vi "Laser Rough Cutting.vi"(0 "configuration file path":path caption="production information", 1 "rough cutting msic":T1) -> ()   [LabVIEW 2018]
uses:
  Ctl.xio/rough cutting msic ctl.ctl
  SubVIS.xio/DataSocket/DataSocket_Tags.ctl
  Ctl.xio/part type.ctl
  SubVIS.xio/Creat Write List VI's/DefCtrl/Station.ctl
  <vilib>/Utility/file.llb/Read From Spreadsheet File (string).vi
  SubVIS.xio/DataSocket/Write PLC Vars/Write Bool Var in.vi
  SubVIS.xio/DataSocket/Read PLC Vars/Read String Var.vi
  SubVIS.xio/DataSocket/Write PLC Vars/Write String Var in.vi
  SubVIS.xio/DataSocket/Write PLC Vars/Write Dbl Var in.vi
  SubVIS.xio/DataSocket/Read PLC Vars/Read Bool Var.vi
panel:
  out "error out 2":errorcluster caption="error out"
  in  "SQL information":string
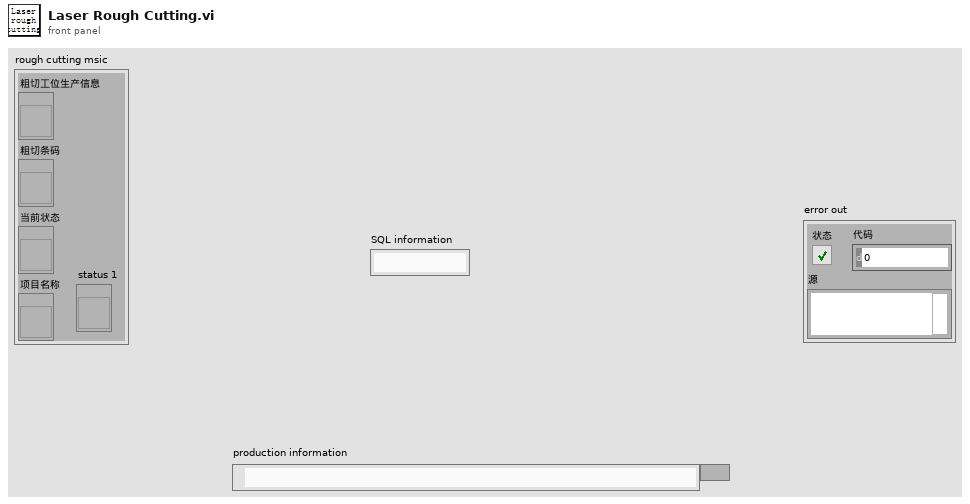
[diagram p1: front panel]
types:
  T1 = cluster{"粗切工位生产信息":refnum<vi>, "粗切条码":refnum<vi>, "当前状态":refnum<vi>, "项目名称":refnum<vi>, "status 1":refnum<vi>}
  T2 = typedef "Station.ctl" = enum16{"粗切工位", "热处理工位", "精切工位", "PDF焊接工位", "打凹点预载力工位", "收卷工位", "EOL工位"}
  T3 = typedef "rough cutting msic ctl.ctl" = cluster{"configuration file path":path, "DsOut":T4[], "scanner coms or ip":string, "BarCode":string, "scanner resource name out":refnum<visa-resource-name>, "Hopper car information":cluster{"Hopper car code":string, "Hopper car No":string, "plate No":string}, "pallet.produced number":i32, "SQL information":string, "Database":string[], "Serial number":i32, "database path":path, "rough cutting msic":cluster{"production info":refnum<vi>, "code":refnum<vi>, "status":refnum<vi>, "part type":refnum<vi>, "status":refnum<vi>}, "Part type":T5, "scanner ip ID":refnum<k5>, "Number of scans ":u8, "Incoming code":string, "Cut file":string, "Process code":string}
  T4 = typedef "DataSocket_Tags.ctl" = cluster{"Ds ID":refnum<k13>, "Tag":string}
  T5 = typedef "part type.ctl" = cluster{"Part type":string, "Material code":string, "Part number":string, "Supplier code":string, "Line code":string, "Customer code":string, "Color code":string, "Upper limit":i32, "Temperature":string, "Tot time":string, "EOL stations":string}
  T6 = cluster{"Hopper car code":string, "Hopper car No":string, "plate No":string}
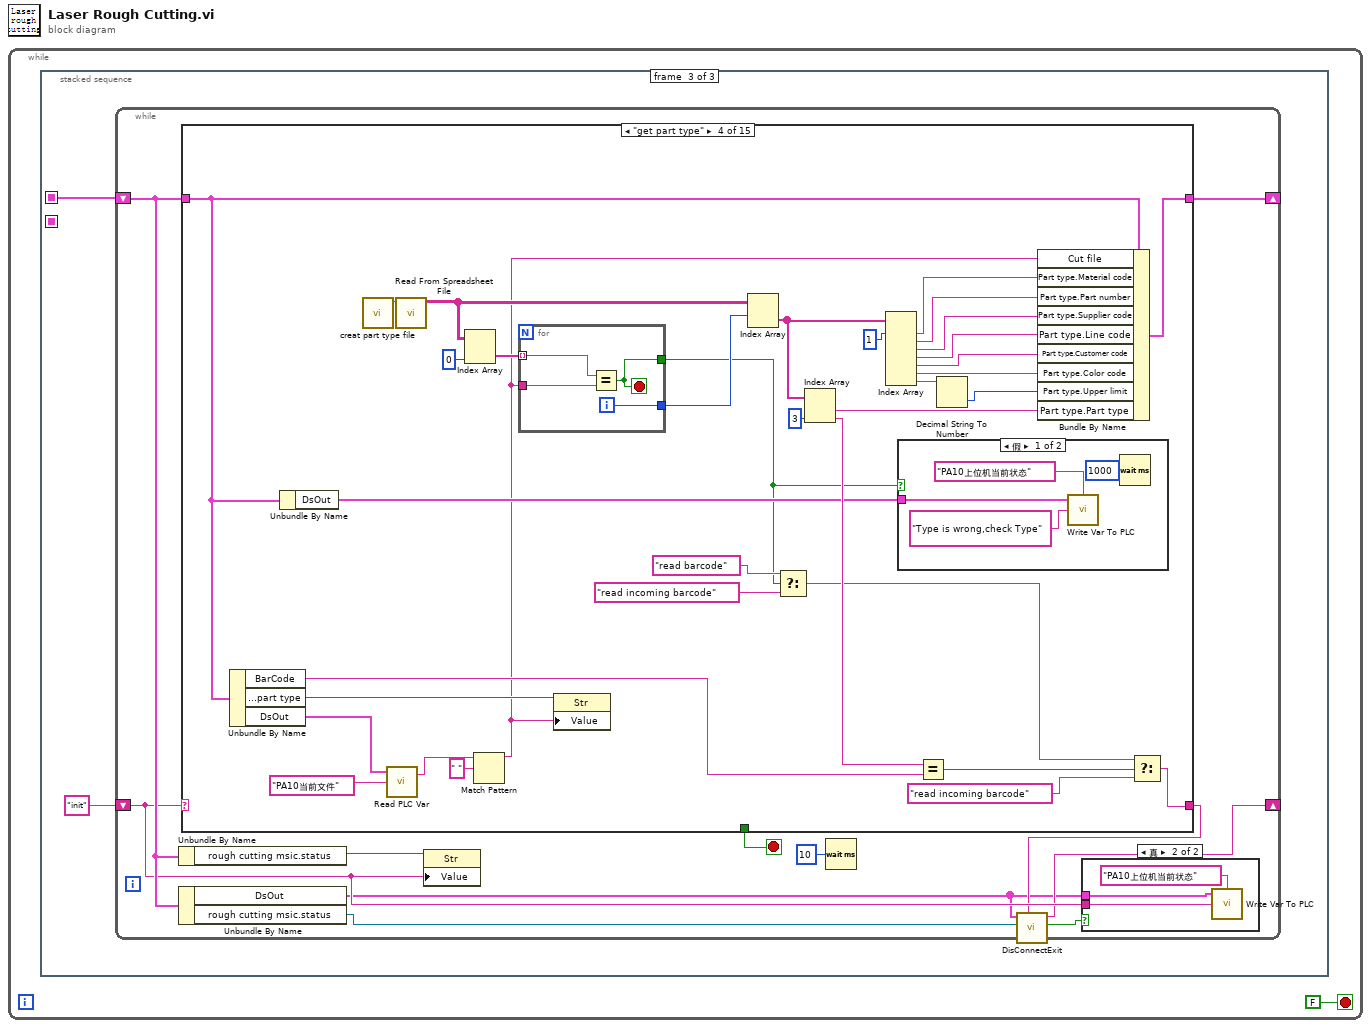
[diagram p0: block diagram]
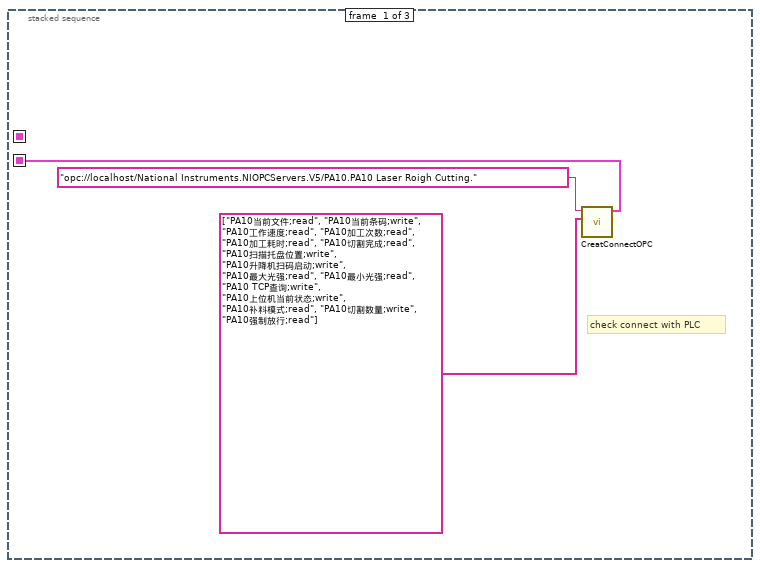
[diagram p2: hidden frame]
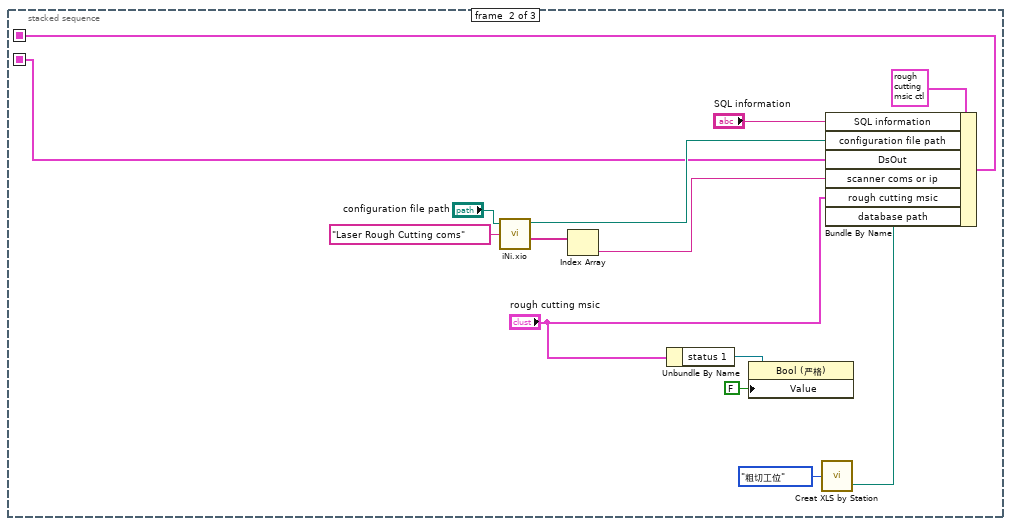
[diagram p3: hidden frame]
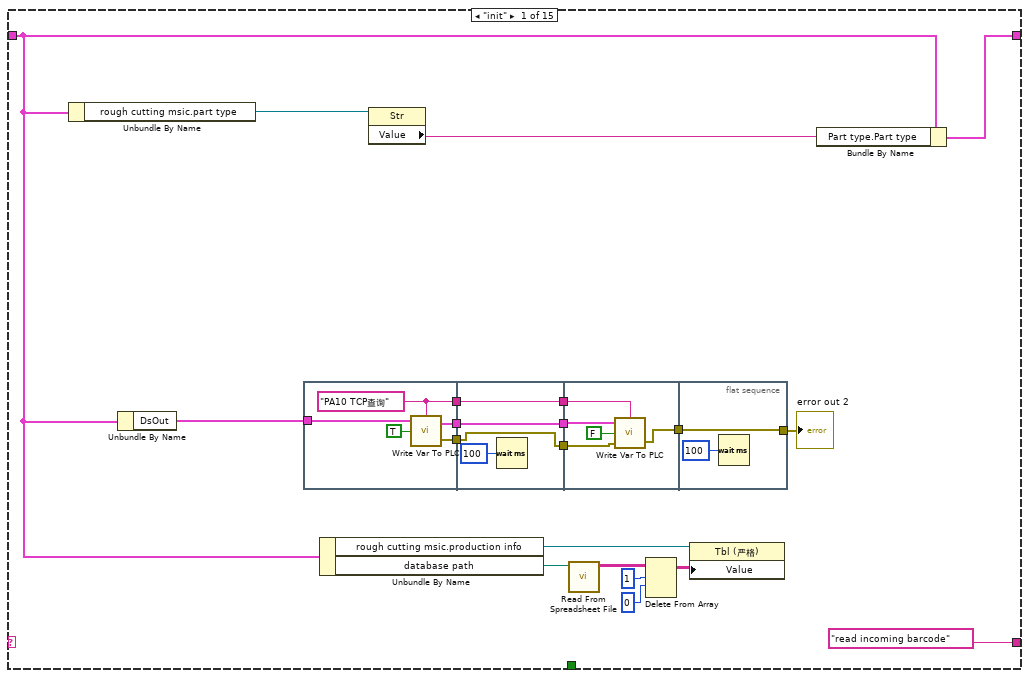
[diagram p5: hidden frame]
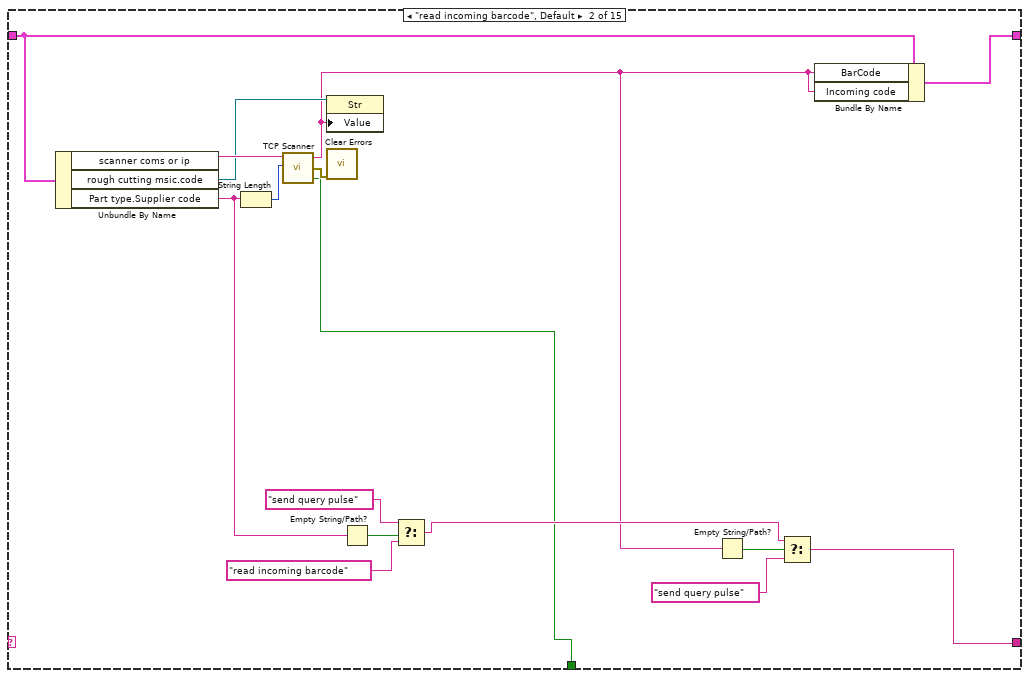
[diagram p6: hidden frame]
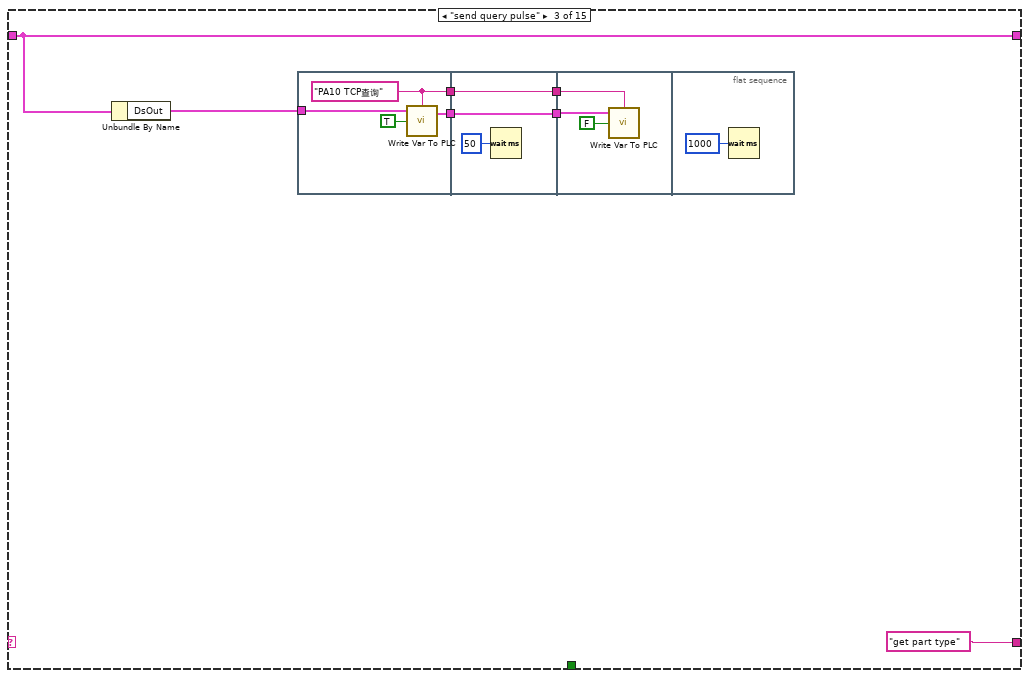
[diagram p7: hidden frame]
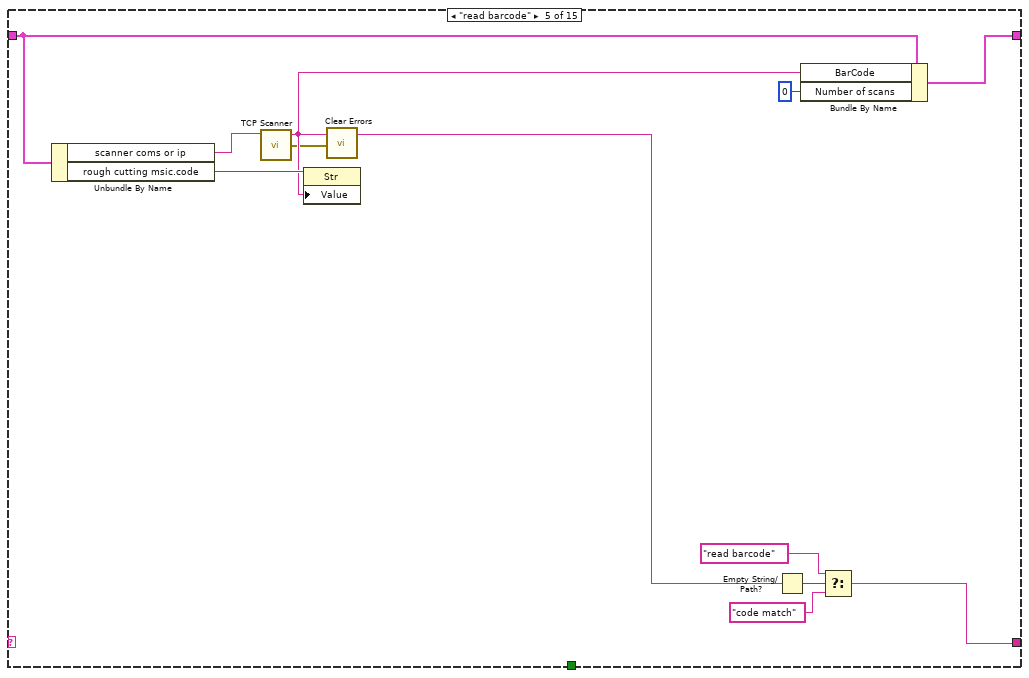
[diagram p9: hidden frame]
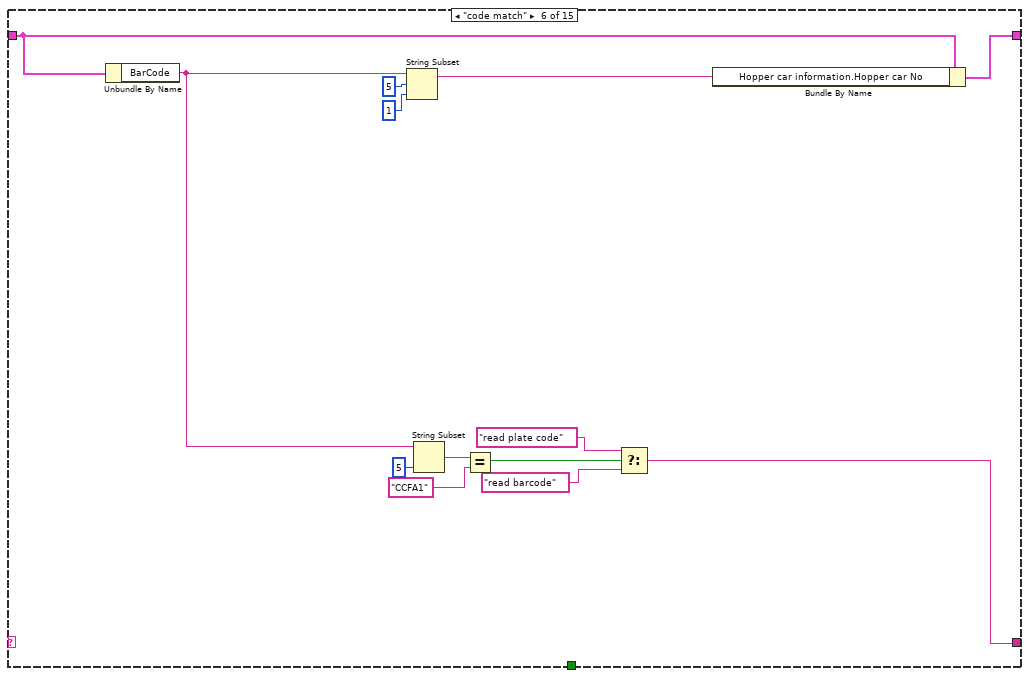
[diagram p10: hidden frame]
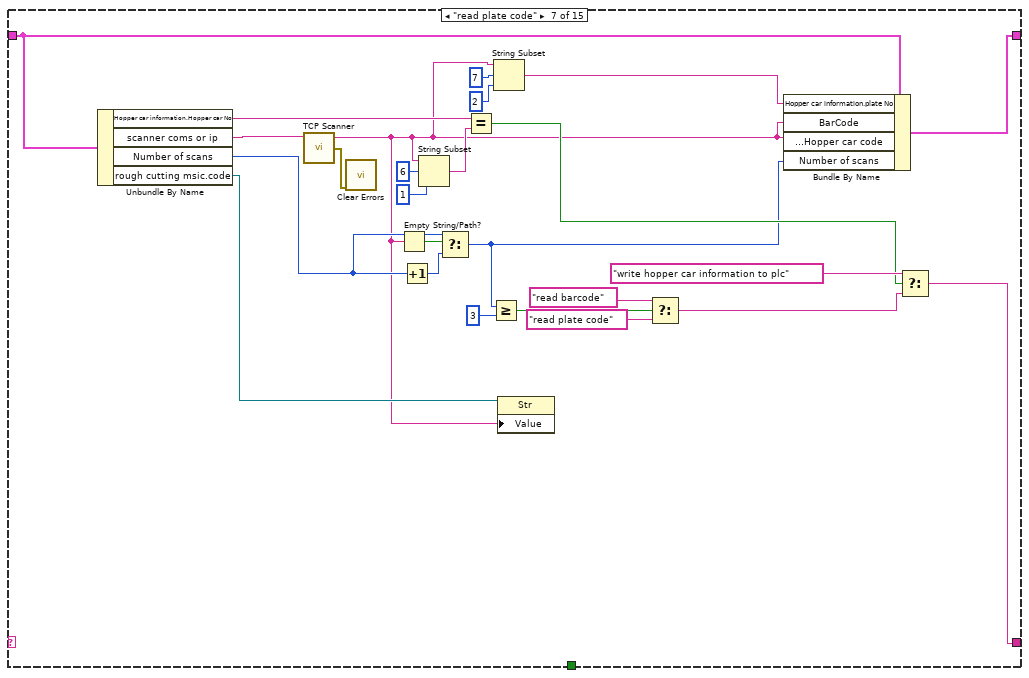
[diagram p11: hidden frame]
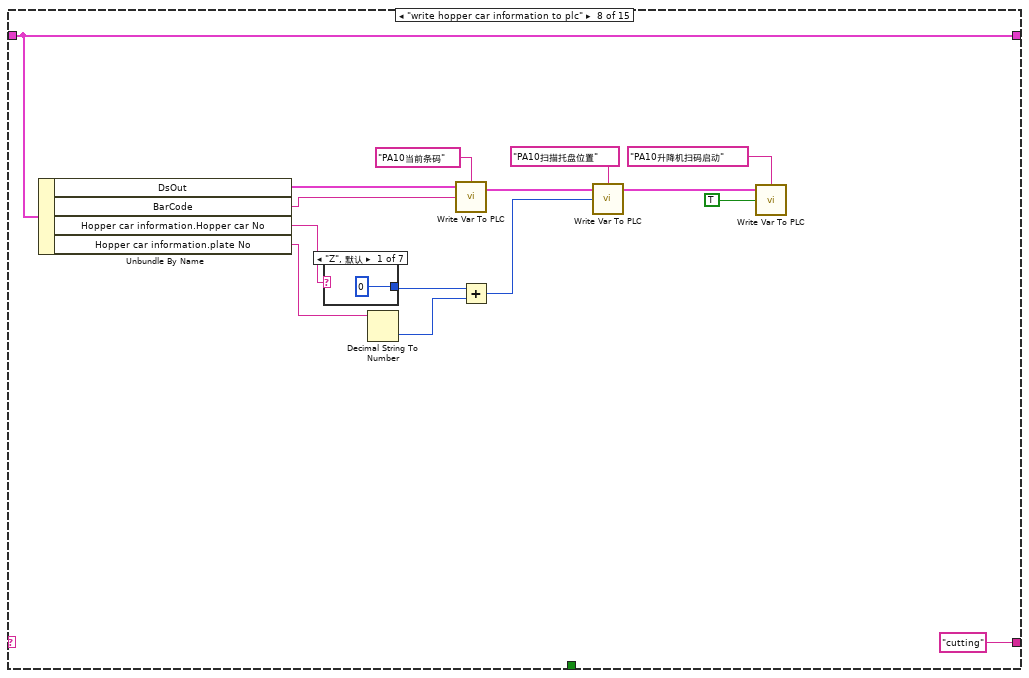
[diagram p12: hidden frame]
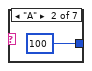
[diagram p13: hidden frame]
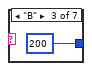
[diagram p14: hidden frame]
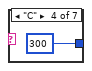
[diagram p15: hidden frame]
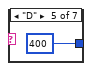
[diagram p16: hidden frame]
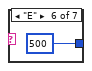
[diagram p17: hidden frame]
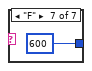
[diagram p18: hidden frame]
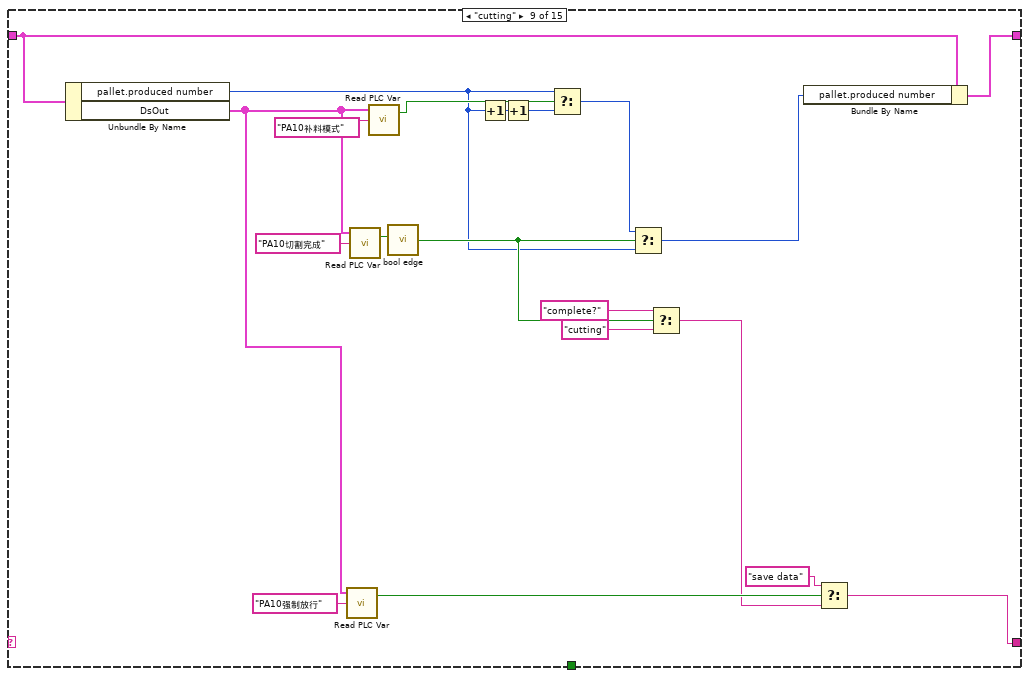
[diagram p19: hidden frame]
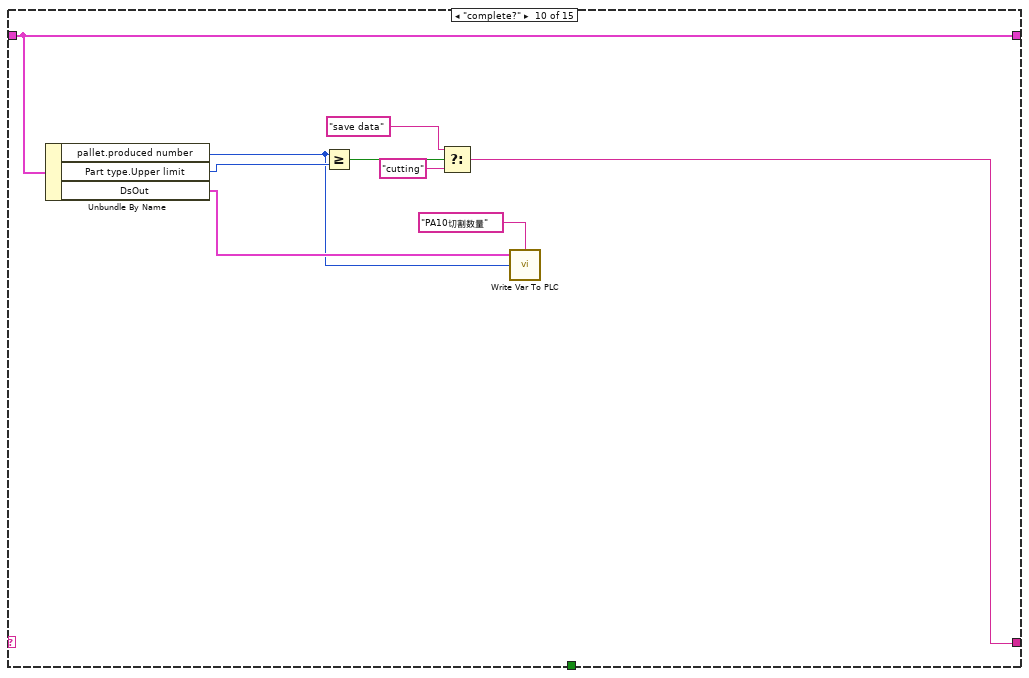
[diagram p20: hidden frame]
diagram:
  n1 = while {
    stop <- FALSE stop-if-true
    n2 = stacked-sequence {
      seq-local: [_ w11 _] -> [_ _ w19]
      seq-local: [w3 _ _] -> [_ w8 _]
      frame #0 {
        # "check connect with PLC"
        n3 = call "CreatConnectOPC.vi"("All Tags"=string[] ["PA10当前文件;read", "PA10当前条码;write", "PA10工作速度;read", "PA10加工次数;read", "PA10加工耗时;read", "PA10切割完成;read", "PA10扫描托盘位置;write", "PA10升降机扫码启动;write", "PA10最大光强;read", "PA10最小光强;read", "PA10 TCP查询;write", "PA10上位机当前状态;write", "PA10补料模式;read", "PA10切割数量;write", "PA10强制放行;read"], "URL"="opc://localhost/National Instruments.NIOPCServers.V5/PA10.PA10 Laser Roigh Cutting.") -> ("DsOut"=w3:T4[])  [unwired: 9 in]
      }
      frame #1 {
        n4 = call "iNi.xio.vi"("configuration file path"="configuration file path", "Sections"="Laser Rough Cutting coms") -> ("configuration file path"=w18:path, "Values"=w16:string[])  [unwired: 1 in, 3 out]
        n5 = Index Array(array=w16) -> (element=w15:string)  [unwired: 1 in]
        n6 = Unbundle By Name("rough cutting msic") -> ("status 1"=w6:refnum<vi>)
        n7 = property class="Bool (严格)"(reference=w6, "Value"=FALSE ("值")) -> ()  [unwired: 1 in, 2 out]
        n8 = call "Creat XLS by Station.vi"("staiton"=Station."粗切工位") -> ("new file path (Not A Path if cancelled)"=w10:path)  [unwired: 5 in]
        n9 = Bundle By Name(cluster=T3 {"configuration file path"=path "", "DsOut"=[], "scanner coms or ip"="", "BarCode"="", "scanner resource name out"="", "Hopper car information"={"Hopper car code"="", "Hopper car No"="", "plate No"=""}, "pallet.produced number"=0, "SQL information"="", "Database"=[], "Serial number"=0, "database path"=path "", "rough cutting msic"={"production info"=refnum, "code"=refnum, "status"=refnum, "part type"=refnum, "status"=refnum}, "Part type"={"Part type"="", "Material code"="", "Part number"="", "Supplier code"="", "Line code"="", "Customer code"="", "Color code"="", "Upper limit"=0, "Temperature"="", "Tot time"="", "EOL stations"=""}, "scanner ip ID"=refnum, "Number of scans "=0, "Incoming code"="", "Cut file"="", "Process code"=""} ("rough cutting msic"), "SQL information"="SQL information", "configuration file path"=w18, "DsOut"=w8, "scanner coms or ip"=w15, "rough cutting msic"="rough cutting msic", "database path"=w10) -> (w11:T3)
      }
      frame #2 {
        n10 = while {
          shift-right: [w31] -> _
          shift-left: w19 -> [w28]
          shift-right: [w24] -> _
          shift-left: "init" ("event") -> [w27]
          stop <- w26 stop-if-true
          n11 = Unbundle By Name(w28) -> ("rough cutting msic.status"=w29:refnum<vi>)
          n12 = Unbundle By Name(w28) -> ("DsOut"=w21:T4[], "rough cutting msic.status"=w23:refnum<vi>)
          n13 = case shown="\"get part type\"" w27 {
            tunnel: w28 -> [w41 w83 w88 w108 w156 w160 w189 w198 w236 w242 w256 w274 w282 w289 w299]
            tunnel: [w54 w86 w88 w139 w155 w168 w188 w198 w238 w242 w258 w275 w282 w294 w299] -> w31
            tunnel: ["read incoming barcode" w78 "get part type" ("f") w132 w151 w166 w191 "cutting" ("event") w222 w245 "database write" ("f") "updata display" ("f") "reset" ("f") "read incoming barcode" ("f") "Exit" ("event")] -> w25
            tunnel: [_ w71 _ _ _ _ _ _ _ _ _ _ _ _ TRUE] -> w26
            frame "init" {
              n14 = Unbundle By Name(w41) -> ("rough cutting msic.part type"=w52:refnum<vi>)
              n15 = Unbundle By Name(w41) -> ("DsOut"=w46:T4[])
              n16 = flat-sequence {
                tunnel: w46 -> [w59]
                tunnel: [w57] -> w50
                tunnel: [w56] -> w49
                tunnel: [w55] -> w37
                tunnel: w50 -> [w62]
                tunnel: [w62] -> w48
                tunnel: w49 -> [w61]
                tunnel: [w61] -> w47
                tunnel: [w60] -> w38
                tunnel: w37 -> [w60]
                tunnel: w48 -> [w68]
                tunnel: w47 -> [w66]
                tunnel: w38 -> [w65]
                tunnel: [w64] -> w36
                tunnel: [w69] -> w35
                tunnel: w36 -> [w69]
                frame #0 {
                  w56 = "PA10 TCP查询" ("Tag IN")
                  n17 = call-poly "Write Var To PLC.vi"("Tag IN"=w56, "Bool Var in"=TRUE, "Ds PLCTags IN"=w59) -> ("error out"=w55:errorcluster, "Ds PLCTags OUT"=w57:T4[])  [unwired: 1 in]
                }
                frame #1 {
                  n18 = Wait (ms)(milliseconds to wait=u32 100 ("等待时间（毫秒）")) -> ()  [unwired: 1 out]
                }
                frame #2 {
                  n19 = call-poly "Write Var To PLC.vi"("Tag IN"=w66, "错误输入（无错误）"=w65, "Bool Var in"=FALSE, "Ds PLCTags IN"=w68) -> ("error out"=w64:errorcluster)  [unwired: 1 out]
                }
                frame #3 {
                  n20 = Wait (ms)(milliseconds to wait=u32 100 ("等待时间（毫秒）")) -> ()  [unwired: 1 out]
                }
              }
              n21 = Unbundle By Name(w41) -> ("rough cutting msic.production info"=w45:refnum<vi>, "database path"=w44:path)
              n22 = property class="Str"(reference=w52) -> ("Value"=w51:string)  [unwired: 1 in, 2 out]
              n23 = call-poly <vilib>:"Read From Spreadsheet File.vi"("file path (dialog if empty)"=w44) -> ("all rows"=w40:string[][])  [unwired: 6 in, 4 out]
              n24 = Delete From Array(array=w40, length=1 ("长度"), index (row)=0 ("索引 (行)")) -> (array with subset deleted=w39:string[][])  [unwired: 1 in, 1 out]
              n25 = property class="Tbl (严格)"(reference=w45, "Value"=w39) -> ()  [unwired: 1 in, 2 out]
              n26 = Bundle By Name(cluster=w41, "Part type.Part type"=w51) -> (w54:T3)
              "error out 2" <- w35
            }
            frame "read incoming barcode", Default {
              n27 = Unbundle By Name(w83) -> ("scanner coms or ip"=w85:string, "rough cutting msic.code"=w84:refnum<vi>, "Part type.Supplier code"=w76:string)
              n28 = String Length(string=w76) -> (length=w82:i32)
              n29 = call "TCP Scanner.vi"("byte of read(9)"=w82, "ip"=w85) -> ("status"=w71:bool, "错误输出"=w81:errorcluster, "Barcode"=w72:string)  [unwired: 2 in]
              n30 = property class="Str"(reference=w84, "Value"=w72) -> ()  [unwired: 1 in, 2 out]
              n31 = call <vilib>:"Clear Errors.vi"("error in (no error)"=w81) -> ()  [unwired: 5 in, 2 out]
              n32 = Empty String/Path?(string/path=w76) -> (empty?=w77:bool)
              n33 = Select(t="send query pulse" ("f"), s=w77, f="read incoming barcode") -> (s? t:f=w73:string)
              n34 = Empty String/Path?(string/path=w72) -> (empty?=w80:bool)
              n35 = Select(t=w73, s=w80, f="send query pulse") -> (s? t:f=w78:string)
              n36 = Bundle By Name(cluster=w83, "BarCode"=w72, "Incoming code"=w72) -> (w86:T3)
            }
            frame "send query pulse" {
              n37 = Unbundle By Name(w88) -> ("DsOut"=w89:T4[])
              n38 = flat-sequence {
                tunnel: w89 -> [w97]
                tunnel: [w95] -> w93
                tunnel: [w94] -> w92
                tunnel: w93 -> [w99]
                tunnel: [w99] -> w91
                tunnel: w92 -> [w98]
                tunnel: [w98] -> w90
                tunnel: w91 -> [w103]
                tunnel: w90 -> [w101]
                frame #0 {
                  w94 = "PA10 TCP查询" ("Tag IN")
                  n39 = call-poly "Write Var To PLC.vi"("Tag IN"=w94, "Bool Var in"=TRUE, "Ds PLCTags IN"=w97) -> ("Ds PLCTags OUT"=w95:T4[])  [unwired: 1 in, 1 out]
                }
                frame #1 {
                  n40 = Wait (ms)(milliseconds to wait=u32 50 ("等待时间（毫秒）")) -> ()  [unwired: 1 out]
                }
                frame #2 {
                  n41 = call-poly "Write Var To PLC.vi"("Tag IN"=w101, "Bool Var in"=FALSE, "Ds PLCTags IN"=w103) -> ()  [unwired: 1 in, 2 out]
                }
                frame #3 {
                  n42 = Wait (ms)(milliseconds to wait=u32 1000 ("等待时间（毫秒）")) -> ()  [unwired: 1 out]
                }
              }
            }
            frame "get part type" {
              n43 = Unbundle By Name(w108) -> ("BarCode"=w114:string, "rough cutting msic.part type"=w115:refnum<vi>, "DsOut"=w122:T4[])
              n44 = Unbundle By Name(w108) -> ("DsOut"=w107:T4[])
              n45 = call "creat part type file.vi"() -> ("new file path (Not A Path if cancelled)"=w133:path)  [unwired: 11 in]
              n46 = call-poly "Read PLC Var.vi"("Tag IN"="PA10当前文件", "Ds PLCTags IN"=w122) -> ("String Var out"=w117:string)  [unwired: 1 in, 1 out]
              n47 = call-poly <vilib>:"Read From Spreadsheet File.vi"("file path (dialog if empty)"=w133) -> ("all rows"=w135:string[][])  [unwired: 6 in, 4 out]
              n48 = Index Array(array=w135, index (col)=0 ("禁用的索引 (列)")) -> (element=w136:string[])  [unwired: 1 in]
              n49 = Match Pattern(string=w117, regular expression=" " ("正则表达式")) -> (before substring=w105:string)  [unwired: 1 in, 3 out]
              n50 = for {
                tunnel: w136 -> [w145] mode=indexing
                tunnel: [w147] -> w134
                tunnel: w105 -> [w146]
                tunnel: [w144] -> w106
                i -> [w147]
                stop <- w144 stop-if-true
                n51 = Equal?(x=w145, y=w146) -> (x = y?=w144:bool)
              }
              n52 = property class="Str"(reference=w115, "Value"=w105) -> ()  [unwired: 1 in, 2 out]
              n53 = Index Array(array=w135, index (row)=w134) -> (element=w121:string[])  [unwired: 1 in]
              n54 = Select(t="read barcode", s=w106, f="read incoming barcode") -> (s? t:f=w109:string)
              n55 = Index Array(array=w121, index #2=3 ("索引")) -> (element #1=w119:string, element #2=w113:string)  [unwired: 1 in]
              n56 = Index Array(array=w121, index #1=1 ("索引")) -> (element #1=w130:string, element #2=w129:string, element #3=w128:string, element #4=w127:string, element #5=w126:string, element #6=w125:string, element #7=w124:string)  [unwired: 6 in]
              n57 = case shown="假" w106 {
                tunnel: w107 -> [w143 _]
                frame False {
                  n58 = call-poly "Write Var To PLC.vi"("Tag IN"="PA10上位机当前状态", "String Var in"="Type is wrong,check Type", "Ds PLCTags IN"=w143) -> ()  [unwired: 1 in, 2 out]
                  n59 = Wait (ms)(milliseconds to wait=u32 1000 ("等待时间（毫秒）")) -> ()  [unwired: 1 out]
                }
                frame True {
                }
              }
              n60 = Equal?(x=w113, y=w114) -> (x = y?=w120:bool)
              n61 = Decimal String To Number(string=w124) -> (number=w131:i32)  [unwired: 2 in, 1 out]
              n62 = Bundle By Name(cluster=w108, "Cut file"=w105, "Part type.Material code"=w130, "Part type.Part number"=w129, "Part type.Supplier code"=w128, "Part type.Line code"=w127, "Part type.Customer code"=w126, "Part type.Color code"=w125, "Part type.Upper limit"=w131, "Part type.Part type"=w119) -> (w139:T3)
              n63 = Select(t=w109, s=w120, f="read incoming barcode") -> (s? t:f=w132:string)
            }
            frame "read barcode" {
              n64 = Unbundle By Name(w156) -> ("scanner coms or ip"=w158:string, "rough cutting msic.code"=w157:refnum<vi>)
              n65 = call "TCP Scanner.vi"("ip"=w158) -> ("错误输出"=w149:errorcluster, "Barcode"=w150:string)  [unwired: 3 in, 1 out]
              n66 = property class="Str"(reference=w157, "Value"=w150) -> ()  [unwired: 1 in, 2 out]
              n67 = call <vilib>:"Clear Errors.vi"("error in (no error)"=w149) -> ()  [unwired: 5 in, 2 out]
              n68 = Empty String/Path?(string/path=w150) -> (empty?=w154:bool)
              n69 = Bundle By Name(cluster=w156, "BarCode"=w150, "Number of scans"=u8 0) -> (w155:T3)
              n70 = Select(t="read barcode", s=w154, f="code match") -> (s? t:f=w151:string)
            }
            frame "code match" {
              n71 = Unbundle By Name(w160) -> ("BarCode"=w159:string)
              n72 = String Subset(string=w159, offset (0)=5 ("偏移量(0)"), length (rest)=1 ("长度（剩余）")) -> (substring=w162:string)
              n73 = String Subset(string=w159, length (rest)=5 ("长度（剩余）")) -> (substring=w163:string)  [unwired: 1 in]
              n74 = Equal?(x=w163, y="CCFA1") -> (x = y?=w167:bool)
              n75 = Select(t="read plate code" ("event"), s=w167, f="read barcode" ("event")) -> (s? t:f=w166:string)
              n76 = Bundle By Name(cluster=w160, "Hopper car information.Hopper car No"=w162) -> (w168:T3)
            }
            frame "read plate code" {
              n77 = Unbundle By Name(w189) -> ("Hopper car information.Hopper car No"=w193:string, "scanner coms or ip"=w196:string, "Number of scans"=w179:u8, "rough cutting msic.code"=w176:refnum<vi>)
              n78 = call "TCP Scanner.vi"("ip"=w196) -> ("错误输出"=w181:errorcluster, "Barcode"=w173:string)  [unwired: 3 in, 1 out]
              n79 = call <vilib>:"Clear Errors.vi"("error in (no error)"=w181) -> ()  [unwired: 5 in, 2 out]
              n80 = Empty String/Path?(string/path=w173) -> (empty?=w180:bool)
              n81 = Increment(x=w179) -> (x+1=w178:u8)
              n82 = String Subset(string=w173, offset (0)=6 ("偏移量(0)"), length (rest)=1 ("长度（剩余）")) -> (substring=w187:string)
              n83 = Select(t=w179, s=w180, f=w178) -> (s? t:f=w177:u8)
              n84 = Equal?(x=w193, y=w187) -> (x = y?=w190:bool)
              n85 = Greater Or Equal?(x=w177, y=u8 3) -> (x >= y?=w185:bool)
              n86 = String Subset(string=w173, offset (0)=7 ("偏移量(0)"), length (rest)=2 ("长度（剩余）")) -> (substring=w172:string)
              n87 = property class="Str"(reference=w176, "Value"=w173) -> ()  [unwired: 1 in, 2 out]
              n88 = Select(t="read barcode" ("event"), s=w185, f="read plate code" ("event")) -> (s? t:f=w182:string)
              n89 = Bundle By Name(cluster=w189, "Hopper car information.plate No"=w172, "BarCode"=w173, "Hopper car information.Hopper car code"=w173, "Number of scans"=w177) -> (w188:T3)
              n90 = Select(t="write hopper car information to plc" ("event"), s=w190, f=w182) -> (s? t:f=w191:string)
            }
            frame "write hopper car information to plc" {
              n91 = Unbundle By Name(w198) -> ("DsOut"=w201:T4[], "BarCode"=w200:string, "Hopper car information.Hopper car No"=w211:string, "Hopper car information.plate No"=w210:string)
              n92 = case shown="\"Z\", 默认" w211 {
                tunnel: [0 100 200 300 400 500 600] -> w209
                frame "Z", Default {
                }
                frame "A" {
                }
                frame "B" {
                }
                frame "C" {
                }
                frame "D" {
                }
                frame "E" {
                }
                frame "F" {
                }
              }
              n93 = Decimal String To Number(string=w210) -> (number=w208:i32)  [unwired: 2 in, 1 out]
              n94 = call-poly "Write Var To PLC.vi"("Tag IN"="PA10当前条码", "String Var in"=w200, "Ds PLCTags IN"=w201) -> ("Ds PLCTags OUT"=w202:T4[])  [unwired: 1 in, 1 out]
              n95 = Add(x=w209, y=w208) -> (x+y=w206:i32)
              n96 = call-poly "Write Var To PLC.vi"("Tag IN"="PA10扫描托盘位置", "Dbl Var in"=w206, "Ds PLCTags IN"=w202) -> ("Ds PLCTags OUT"=w205:T4[])  [unwired: 1 in, 1 out]
              n97 = call-poly "Write Var To PLC.vi"("Tag IN"="PA10升降机扫码启动", "Bool Var in"=TRUE, "Ds PLCTags IN"=w205) -> ()  [unwired: 1 in, 2 out]
            }
            frame "cutting" {
              n98 = Unbundle By Name(w236) -> ("pallet.produced number"=w220:i32, "DsOut"=w225:T4[])
              n99 = call-poly "Read PLC Var.vi"("Tag IN"="PA10强制放行", "Ds PLCTags IN"=w225) -> ("Bool Var out"=w224:bool)  [unwired: 1 in, 1 out]
              n100 = call-poly "Read PLC Var.vi"("Tag IN"="PA10切割完成", "Ds PLCTags IN"=w225) -> ("Bool Var out"=w231:bool)  [unwired: 1 in, 1 out]
              n101 = call-poly "Read PLC Var.vi"("Tag IN"="PA10补料模式", "Ds PLCTags IN"=w225) -> ("Bool Var out"=w229:bool)  [unwired: 1 in, 1 out]
              n102 = call "bool edge.vi"("bool in"=w231) -> ("true-false"=w235:bool)  [unwired: 6 in, 1 out]
              n103 = Increment(x=w220) -> (x+1=w219:i32)
              n104 = Increment(x=w219) -> (x+1=w228:i32)
              n105 = Select(t=w220, s=w229, f=w228) -> (s? t:f=w227:i32)
              n106 = Select(t=w227, s=w235, f=w220) -> (s? t:f=w237:i32)
              n107 = Select(t="complete?" ("event"), s=w235, f="cutting" ("event")) -> (s? t:f=w223:string)
              n108 = Bundle By Name(cluster=w236, "pallet.produced number"=w237) -> (w238:T3)
              n109 = Select(t="save data" ("event"), s=w224, f=w223) -> (s? t:f=w222:string)
            }
            frame "complete?" {
              n110 = Unbundle By Name(w242) -> ("pallet.produced number"=w240:i32, "Part type.Upper limit"=w247:i32, "DsOut"=w241:T4[])
              n111 = Greater Or Equal?(x=w240, y=w247) -> (x >= y?=w246:bool)
              n112 = Select(t="save data" ("event"), s=w246, f="cutting") -> (s? t:f=w245:string)
              n113 = call-poly "Write Var To PLC.vi"("Tag IN"="PA10切割数量", "Dbl Var in"=w240, "Ds PLCTags IN"=w241) -> ()  [unwired: 1 in, 2 out]
            }
            frame "save data" {
              n114 = Unbundle By Name(w256) -> ("BarCode"=w257:string, "Cut file"=w254:string, "Part type.Part type"=w250:string, "Hopper car information.Hopper car code"=w253:string, "Incoming code"=w248:string)  [unwired: 1 out]
              n115 = call "TimeDate.vi"() -> ("time_Y/M/D S"=w252:string, "time_YMD"=w251:string)  [unwired: 10 in]
              n116 = Concatenate Strings(w250, w253, w252) -> (w249:string)
              n117 = Build Array(w251, w257, w254, w250, w249, w248) -> (w259:string[])
              n118 = Bundle By Name(cluster=w256, "Database"=w259, "Process code"=w249) -> (w258:T3)
              n119 = Wait (ms)(milliseconds to wait=u32 100 ("等待时间（毫秒）")) -> ()  [unwired: 1 out]
            }
            frame "database write" {
              w271 = enum16{"read", "write"}."write" ("write\\read")
              n120 = Unbundle By Name(w274) -> ("configuration file path"=w273:path, "BarCode"=w270:string)
              n121 = Unbundle By Name(w274) -> ("Database"=w261:string[], "Process code"=w262:string)
              n122 = String Subset(string=w270, length (rest)=6 ("长度（剩余）")) -> (substring=w268:string)  [unwired: 1 in]
              n123 = call "Hopper car inf.vi"("write\\read（read)"=w271, "value"=w262, "key"=w270, "path in"=w273) -> ("path out"=w272:path)  [unwired: 6 in, 1 out]
              n124 = Concatenate Strings(w268, "000") -> (w266:string)
              n125 = call "Hopper car inf.vi"("write\\read（read)"=w271, "value"=w262, "key"=w266, "path in"=w272) -> ()  [unwired: 6 in, 2 out]
              n126 = call "Creat XLS by Station.vi"("staiton"=Station."粗切工位", "data in"=w261) -> ("new file path (Not A Path if cancelled)"=w264:path)  [unwired: 4 in]
              n127 = Bundle By Name(cluster=w274, "database path"=w264) -> (w275:T3)
              n128 = Wait (ms)(milliseconds to wait=u32 100 ("等待时间（毫秒）")) -> ()  [unwired: 1 out]
            }
            frame "updata display" {
              n129 = Unbundle By Name(w282) -> ("rough cutting msic.production info"=w284:refnum<vi>, "database path"=w283:path)
              n130 = call-poly <vilib>:"Read From Spreadsheet File.vi"("file path (dialog if empty)"=w283) -> ("all rows"=w281:string[][])  [unwired: 6 in, 4 out]
              n131 = Delete From Array(array=w281, length=1 ("长度"), index (row)=0 ("索引 (行)")) -> (array with subset deleted=w278:string[][])  [unwired: 1 in, 1 out]
              n132 = property class="Tbl (严格)"(reference=w284, "Value"=w278) -> ()  [unwired: 1 in, 2 out]
              n133 = Wait (ms)(milliseconds to wait=u32 100 ("等待时间（毫秒）")) -> ()  [unwired: 1 out]
            }
            frame "reset" {
              n134 = Unbundle By Name(w289) -> ("rough cutting msic.code"=w288:refnum<vi>)
              n135 = property class="Str"(reference=w288, "Value"="" ("值")) -> ()  [unwired: 1 in, 2 out]
              n136 = Bundle By Name(cluster=w289, "Number of scans"=u8 0, "pallet.produced number"=0, "BarCode"="", "Database"=string[] [], "Hopper car information"=T6 {"Hopper car code"="", "Hopper car No"="", "plate No"=""}) -> (w294:T3)
              n137 = Wait (ms)(milliseconds to wait=u32 100 ("等待时间（毫秒）")) -> ()  [unwired: 1 out]
            }
            frame "Exit" {
            }
          }
          n138 = property class="Str"(reference=w29, "Value"=w27) -> ()  [unwired: 1 in, 2 out]
          n139 = Wait (ms)(milliseconds to wait=u32 10 ("等待时间（毫秒）")) -> ()  [unwired: 1 out]
          n140 = call "DisConnectExit.vi"("Event in"=w25, "status"=w23, "Ds PLCTags IN"=w21) -> ("status？"=w22:bool, "Event out"=w24:string)  [unwired: 7 in]
          n141 = case shown="真" w22 {
            tunnel: w27 -> [_ w33]
            tunnel: w21 -> [_ w32]
            frame False {
            }
            frame True {
              n142 = call-poly "Write Var To PLC.vi"("Tag IN"="PA10上位机当前状态", "String Var in"=w33, "Ds PLCTags IN"=w32) -> ()  [unwired: 1 in, 2 out]
            }
          }
        }
      }
    }
  }
